vi "AI 1 Samples FPGA.vi"() -> ()   [LabVIEW 2019]
uses:
  <vilib>/LabVIEW Targets/FPGA/RIO/BlueMoonOnboardIO/nicrio_cRIO-BlueMoonOnboardAi_VoltageRange.ctl
  <vilib>/LabVIEW Targets/FPGA/RIO/BlueMoonOnboardIO/nicrio_cRIO-BlueMoonOnboardAi_TerminalMod.ctl
  <vilib>/rvi/Emulation/niFpgaGetClockAttributes.vi
  <vilib>/rvi/Emulation/niFpgaSctlEmulationGetInTimedLoop.vi
  <vilib>/rvi/Emulation/niFpgaEmulationReportErrorSimple.vi
  <vilib>/rvi/eio/common/nirviEmuTemplateMethod_errors.vi
  <vilib>/rvi/Emulation/niFpgaCriticalErrorInLSC.vi
  <vilib>/eio/EIOMethodNode/EIOMethodNode.xnode
panel:
  in  "A?B":bool
  in  "Triger\nGet":bool
  out "Data":fxp<+/-,24,5>
  in  "Channel Number":u8
  in  "Terminal Mode":T1=1 items=["DIFF", "RSE"]
  in  "Voltage Range":T2 items=["+/- 10V", "+/- 5V", "+/- 2V", "+/- 1V"]
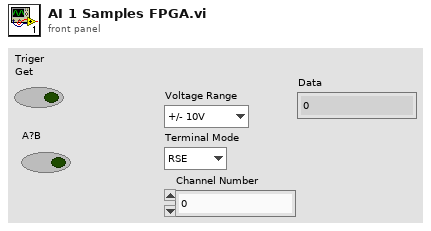
[diagram p1: front panel]
types:
  T1 = typedef "nicrio_cRIO-BlueMoonOnboardAi_TerminalMod.ctl" = u8
  T2 = typedef "nicrio_cRIO-BlueMoonOnboardAi_VoltageRange.ctl" = u8
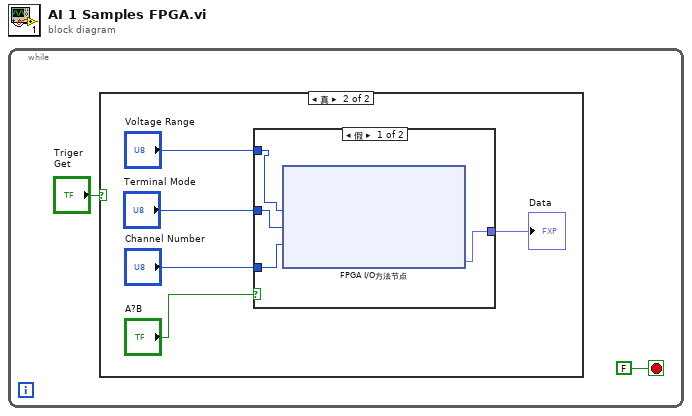
[diagram p0: block diagram]
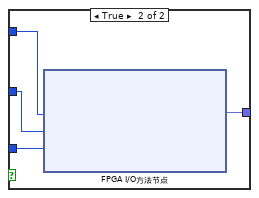
[diagram p3: hidden frame]
diagram:
  n1 = while {
    stop <- FALSE stop-if-true
    n2 = case shown="真" "Triger\nGet" {
      frame False {
      }
      frame True {
        n3 = case shown="假" "A?B" {
          tunnel: "Voltage Range" -> [w11 w15]
          tunnel: "Terminal Mode" -> [w10 w14]
          tunnel: "Channel Number" -> [w9 w13]
          tunnel: [w8 w12] -> w4
          frame False {
            n4 = xnode "FPGA I/O方法节点"("Voltage Range [i + 1]"=w11, "Terminal Mode [i + 1]"=w10, "Channel Number [i + 1]"=w9) -> ("Data [i]"=w8:fxp<+/-,24,5>)  [unwired: 1 in, 1 out]
          }
          frame True {
            n5 = xnode "FPGA I/O方法节点"("Voltage Range [i + 1]"=w15, "Terminal Mode [i + 1]"=w14, "Channel Number [i + 1]"=w13) -> ("Data [i]"=w12:fxp<+/-,24,5>)  [unwired: 1 in, 1 out]
          }
        }
        "Data" <- w4
      }
    }
  }
